vi "PE Get System Name.vi"(8 "error in (no error)":errorcluster, 9 "size":i32, 10 "index":i32, 11 "peHandle":u32) -> (0 "error out":errorcluster, 2 "function return":i32, 3 "name":string)   [LabVIEW 2011, in "libPhyspec.lvlib"]
doc: "PHYSPEC_API PE_STATUS PE_GetSystemName(CPE_HANDLE peHandle, int index, char *name, int size);"
uses:
  libPhyspec.lvlib
  libPhyspec.dll
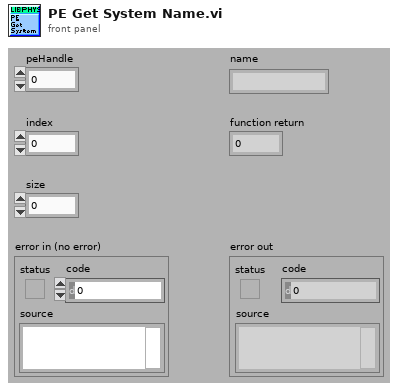
[diagram p1: front panel]
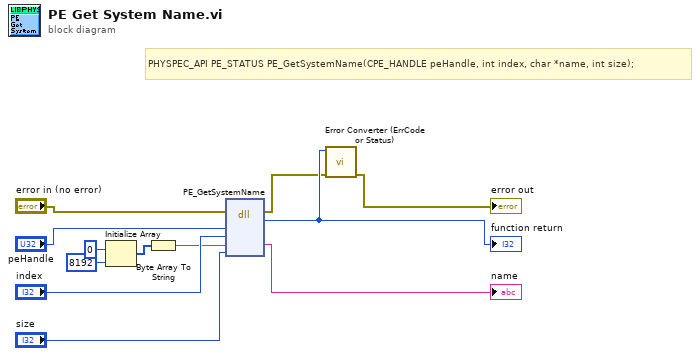
[diagram p0: block diagram]
diagram:
  # "PHYSPEC_API PE_STATUS PE_GetSystemName(CPE_HANDLE peHandle, int index, char *name, int size);"
  n1 = Initialize Array(u8 0 ("element"), 8192 ("dimension size")) -> (w9:u8[])
  n2 = Byte Array To String(unsigned byte array=w9) -> (string=w8:string)
  n3 = dll-call lib="D:/users/nicolas/PHySpec-SDK-1.0.0/Labview-example/libPhyspec/libPhyspec.*" fn="PE_GetSystemName"(error in="error in (no error)", "peHandle"="peHandle", "index"="index", "name"=w8, "size"="size") -> (error out=w2:errorcluster, "return type"=w12:i32, "name"=→"name":string)  [unwired: 5 in, 1 out]
  "function return" <- w12
  n4 = call "Error Converter (ErrCode or Status).vi"("error in (no error)"=w2, "error code"=w12) -> ("error out"=→"error out":errorcluster)  [unwired: 9 in]
